vi "Pre_Pic_XY_Basic.vi"() -> ()   [LabVIEW 2011]
uses:
  <vilib>/Utility/miscctls.llb/LVPoint32TypeDef.ctl
  <vilib>/Utility/miscctls.llb/LVBoundsTypeDef.ctl
panel:
  out "mu08txtChoicePicOriginPoint":T1
  out "TxtChoiceBuf":picture
  out "绘图区域大小":T2
  out "Remain":i32
  out "ColorArray":u32[](array[colorbox])=[16770560, 7995178, 2818039]
  out "mbfTxtChoice":bool[](array[boolean])
  out "Index":i32
  out "StrArray":string[](array[string])=["ValveCold", "ValveHot", "ValvePre", "WaterShot", "ValveBleach", "ValveDry", "ValveMist", "ValveSteam", "ValveChange", "ValveSoftener", "ValveFilter", "ValveActiveWash"]
  out "x-y":T3
  in  "TxtChoice_YScrollBar":i32(c297)
  out "TxtChoice":picture
  out "mu08TextOffsetInit":T4={"X_Offset"=0, "Y_Offset"=0, "TxtHigh"=16, "TxtWidth"=111, "TxtInterval"=16}
  out "Vertical":i32=3
  out "Horizontal":i32=92
  out "数值":i32
  in  "Y":i32(c297)
  in  "X":i32(c297)
  out "X_Y坐标系统":picture
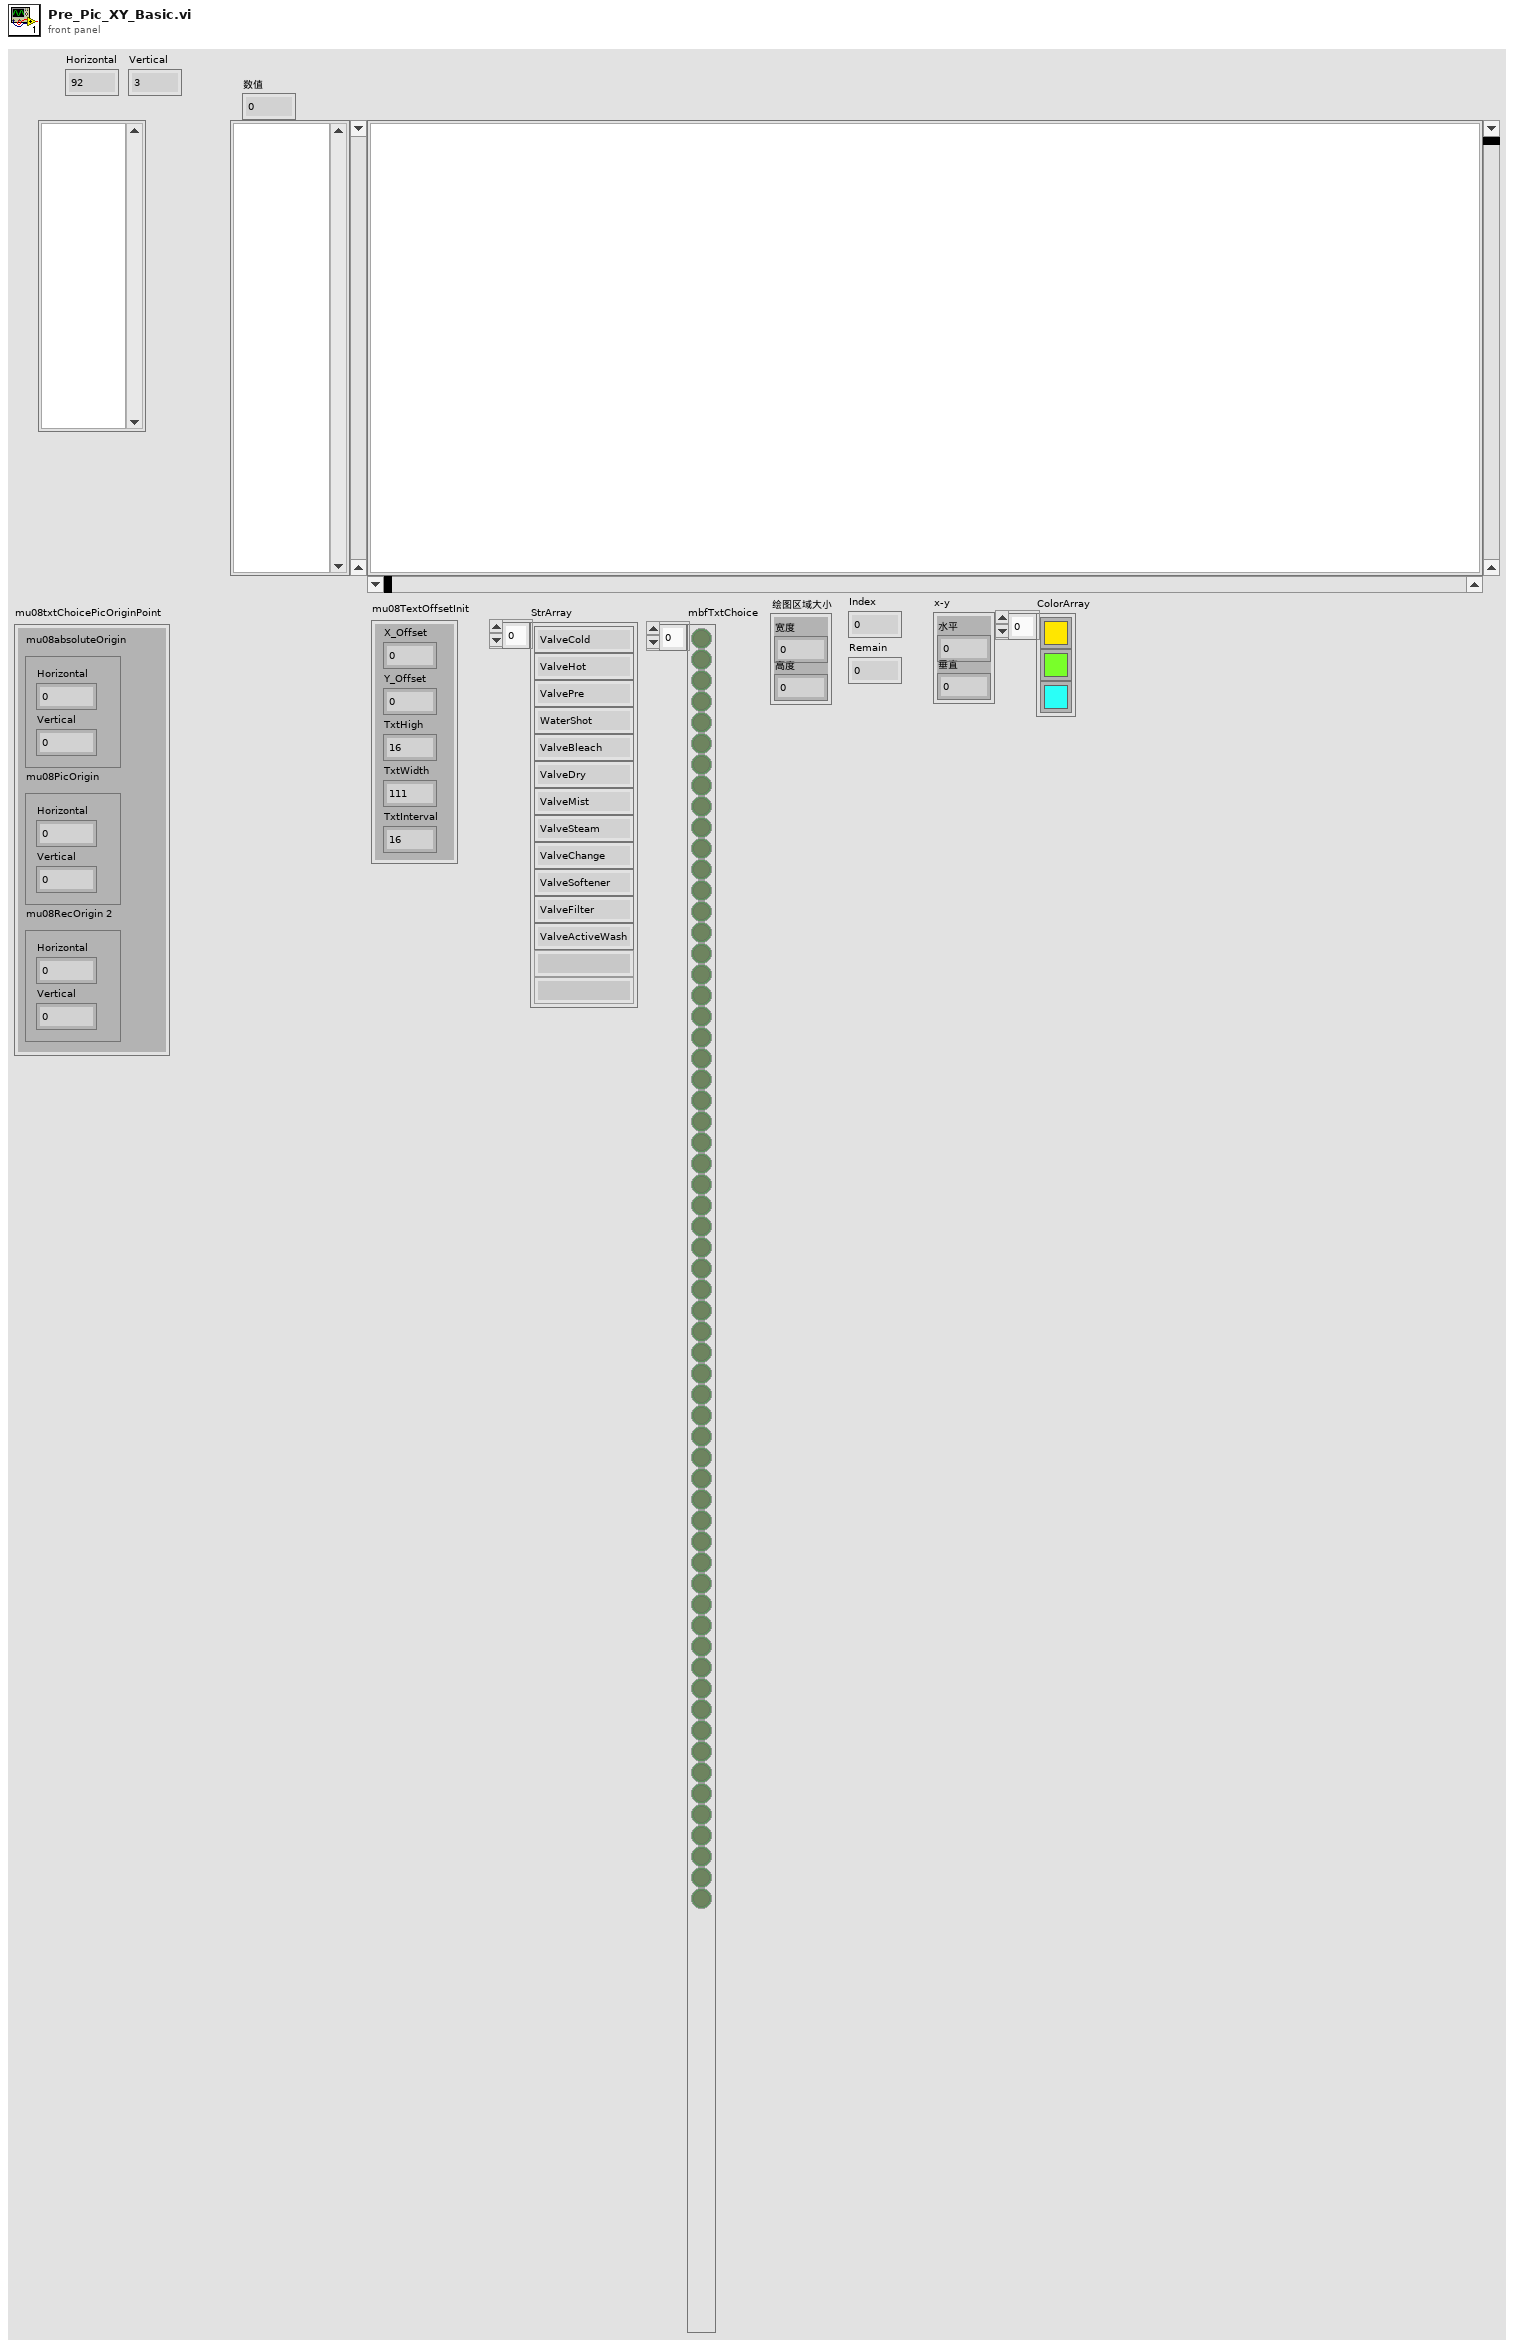
[diagram p1: front panel]
types:
  T1 = cluster{"mu08absoluteOrigin":cluster{"Horizontal":dbl, "Vertical":dbl}, "mu08PicOrigin":cluster{"Horizontal":dbl, "Vertical":dbl}, "mu08RecOrigin 2":cluster{"Horizontal":dbl, "Vertical":dbl}}
  T2 = typedef "LVBoundsTypeDef.ctl" = cluster{"Width":u32, "Height":u32}
  T3 = typedef "LVPoint32TypeDef.ctl" = cluster{"Horizontal":i32, "Vertical":i32}
  T4 = cluster{"X_Offset":u8, "Y_Offset":u8, "TxtHigh":u8, "TxtWidth":u8, "TxtInterval":u8}
  T5 = typedef "LVPositionTypeDef.ctl" = cluster{"Left":i32, "Top":i32}
  T6 = cluster{"Position":T5, cluster{i32, i32}, cluster{i32, i32}}
  T7 = typedef "imagedata.ctl" = cluster{"image type":i32, "image depth":i32, "image":u8[], "mask":u8[], "colors":u32[], "Rectangle":cluster{"left":i16, "top":i16, "right":i16, "bottom":i16}}
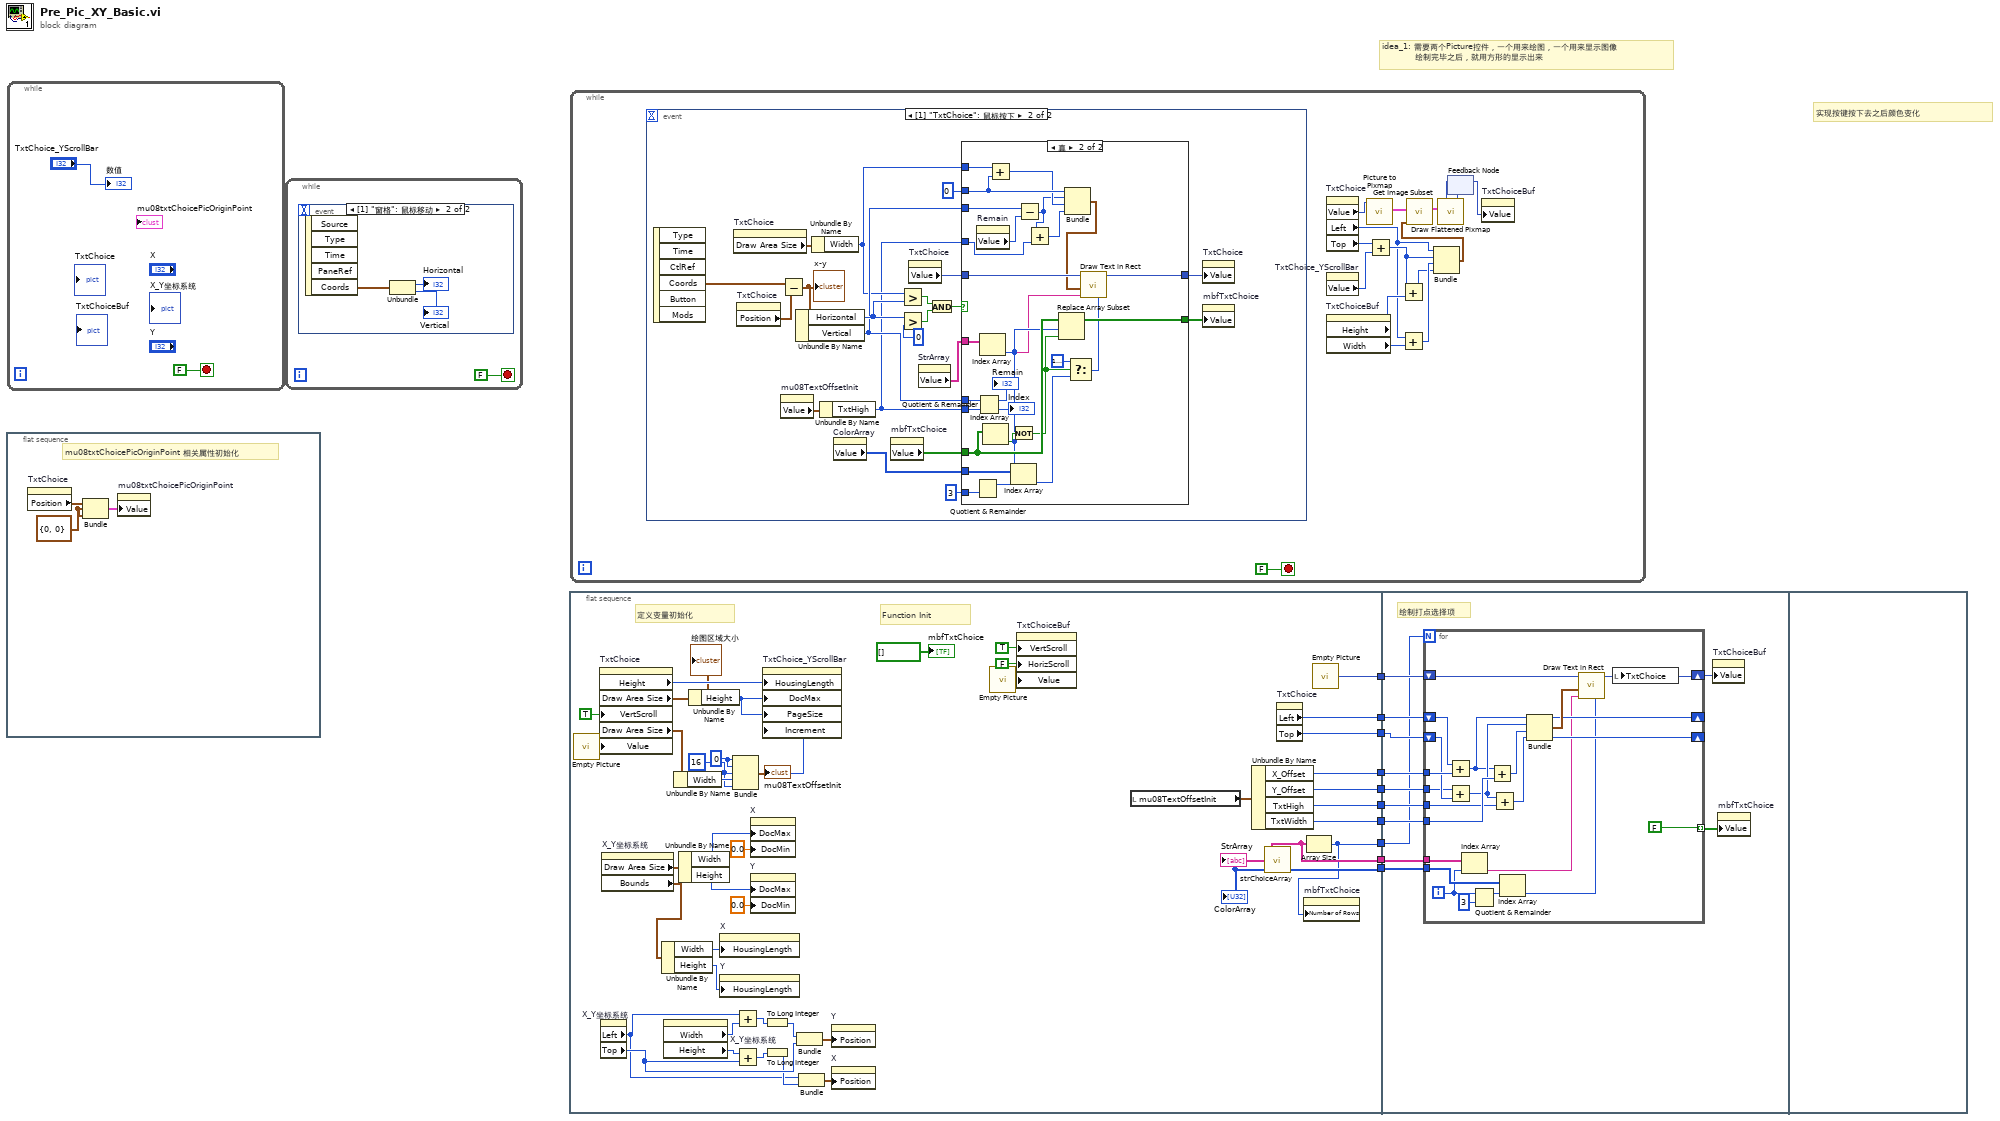
[diagram p0: block diagram]
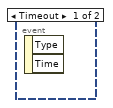
[diagram p2: hidden frame]
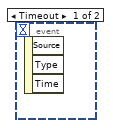
[diagram p4: hidden frame]
diagram:
  # "实现按键按下去之后颜色变化"
  # "idea_1: 需要两个Picture控件，一个用来绘图，一个用来显示图像\n           绘制完毕之后，就用方形的显示出来"
  n1 = flat-sequence {
    frame #0 {
      w12 = cluster{i32, i32} {0, 0}
      # "mu08txtChoicePicOriginPoint 相关属性初始化"
      n2 = property on="TxtChoice" class="Pict"() -> ("Position"=w13:T5)  [unwired: 2 in, 2 out]
      n3 = Bundle("Position"=w13, w12, w12) -> (w11:T6)  [unwired: 1 in]
      n4 = property on="mu08txtChoicePicOriginPoint" class="Clust (严格)"("Value"=w11) -> ()  [unwired: 2 in, 2 out]
    }
  }
  n5 = while {
    stop <- FALSE stop-if-true
    "数值" <- "TxtChoice_YScrollBar"
  }
  n6 = while {
    stop <- FALSE stop-if-true
    n7 = event shown="[1] \"窗格\": 鼠标移动" {
      selector: _ -> [_ _]
      dyn-events: _ -> [_ _]
      timeout: _ -> [_ _]
      event Timeout {
        n8 = event-data() -> ()  [unwired: 1 in, 3 out]
      }
      event Mouse Move {
        n9 = event-data() -> ("Coords"=w19:T3)  [unwired: 1 in, 4 out]
        n10 = Unbundle(w19) -> ("Horizontal"=→"Horizontal":i32, "Vertical"=→"Vertical":i32)
      }
    }
  }
  n11 = flat-sequence {
    tunnel: [w45] -> w10
    tunnel: [w44] -> w9
    tunnel: [w43] -> w8
    tunnel: [w41] -> w7
    tunnel: [w40] -> w6
    tunnel: [w39] -> w5
    tunnel: [w38] -> w4
    tunnel: [w31] -> w3
    tunnel: [w34] -> w2
    tunnel: [w33] -> w1
    tunnel: w10 -> [w74]
    tunnel: w9 -> [w72]
    tunnel: w8 -> [w71]
    tunnel: w7 -> [w73]
    tunnel: w6 -> [w68]
    tunnel: w5 -> [w70]
    tunnel: w4 -> [w69]
    tunnel: w3 -> [w67]
    tunnel: w2 -> [w66]
    tunnel: w1 -> [w65]
    frame #0 {
      w35 = 0
      w23 = 16
      # "Function Init"
      # "定义变量初始化"
      n12 = call "Empty Picture"() -> ("empty picture"=w21:picture)
      n13 = property on="TxtChoice" class="Pict"("VertScroll"=TRUE ("垂直滚动条可见"), "Value"=w21) -> ("Height"=w28:u32, "Draw Area Size"=w27:T2, "Draw Area Size"=w24:T2)  [unwired: 2 in, 2 out]
      "绘图区域大小" <- w27
      n14 = property on="X_Y坐标系统" class="Pict"() -> ("Left"=w49:i32, "Top"=w51:i32)  [unwired: 2 in, 2 out]
      n15 = property on="X_Y坐标系统" class="Pict"() -> ("Draw Area Size"=w62:T2, "Bounds"=w29:T2)  [unwired: 2 in, 2 out]
      n16 = Unbundle By Name(w29) -> ("Width"=w57:u32, "Height"=w56:u32)
      n17 = property on="X_Y坐标系统" class="Pict"() -> ("Width"=w55:u32, "Height"=w54:u32)  [unwired: 2 in, 2 out]
      n18 = Unbundle By Name(w24) -> ("Width"=w37:u32)
      n19 = Unbundle By Name(w62) -> ("Width"=w60:u32, "Height"=w61:u32)
      n20 = Unbundle By Name(w27) -> ("Height"=w26:u32)
      n21 = property on="X" class="Scroll (严格)"("HousingLength"=w57) -> ()  [unwired: 2 in, 2 out]
      n22 = property on="Y" class="Scroll (严格)"("HousingLength"=w56) -> ()  [unwired: 2 in, 2 out]
      n23 = Bundle(w35, w35, w23, "Width"=w37, w23) -> (→"mu08TextOffsetInit":cluster{i32, i32, i32, "Width":u32, i32})  [unwired: 1 in]
      n24 = Add(x=w49, y=w55) -> (x+y=w47:u32)
      n25 = Add(x=w54, y=w51) -> (x+y=w46:u32)
      n26 = property on="X" class="Scroll (严格)"("DocMax"=w60, "DocMin"=0.0 ("滚动范围最小值")) -> ()  [unwired: 2 in, 2 out]
      n27 = property on="Y" class="Scroll (严格)"("DocMax"=w61, "DocMin"=0.0 ("滚动范围最小值")) -> ()  [unwired: 2 in, 2 out]
      n28 = property on="TxtChoice_YScrollBar" class="Scroll (严格)"("HousingLength"=w28, "DocMax"=w26, "PageSize"=w26, "Increment"=w23) -> ()  [unwired: 2 in, 2 out]
      n29 = To Long Integer(number=w47) -> (32bit integer=w53:i32)
      n30 = To Long Integer(number=w46) -> (32bit integer=w50:i32)
      n31 = Bundle(w53, "Top"=w51) -> (w52:cluster{i32, "Top":i32})  [unwired: 1 in]
      n32 = Bundle("Left"=w49, w50) -> (w48:cluster{"Left":i32, i32})  [unwired: 1 in]
      n33 = property on="Y" class="Scroll (严格)"("Position"=w52) -> ()  [unwired: 2 in, 2 out]
      n34 = property on="X" class="Scroll (严格)"("Position"=w48) -> ()  [unwired: 2 in, 2 out]
      n35 = call "Empty Picture"() -> ("empty picture"=w20:picture)
      n36 = property on="TxtChoiceBuf" class="Pict"("VertScroll"=TRUE ("垂直滚动条可见"), "HorizScroll"=FALSE ("水平滚动条可见"), "Value"=w20) -> ()  [unwired: 2 in, 2 out]
      n37 = local read "mu08TextOffsetInit"() -> (w42:T4)
      n38 = Unbundle By Name(w42) -> ("X_Offset"=w41:u8, "Y_Offset"=w40:u8, "TxtHigh"=w38:u8, "TxtWidth"=w39:u8)
      n39 = call "strChoiceArray.vi"() -> ("ColorArray"=w33:u32[], "StrArray"=w34:string[])
      "StrArray" <- w34
      "ColorArray" <- w33
      n40 = property on="TxtChoice" class="Pict"() -> ("Left"=w44:i16, "Top"=w43:i16)  [unwired: 2 in, 2 out]
      n41 = Array Size(array=w34) -> (size(s)=w31:i32)
      n42 = property on="mbfTxtChoice" class="Arr (严格)"("Number of Rows"=w31) -> ()  [unwired: 2 in, 2 out]
      n43 = call "Empty Picture"() -> ("empty picture"=w45:picture)
      "mbfTxtChoice" <- bool[] [] ("mbfTxtChoice")
    }
    frame #1 {
      # "绘制打点选择项"
      n44 = for {
        N: w67 -> [_]
        tunnel: w73 -> [w94]
        tunnel: w70 -> [w91]
        tunnel: w69 -> [w89]
        tunnel: w68 -> [w87]
        shift-right: [w86] -> w63
        shift-left: w74 -> [w95]
        shift-right: [w83] -> _
        shift-left: w72 -> [w93]
        shift-right: [w84] -> _
        shift-left: w71 -> [w92]
        tunnel: w66 -> [w82]
        tunnel: w65 -> [w80]
        tunnel: [FALSE] -> w64 mode=indexing
        i -> [w79]
        n45 = Add(x=w93, y=w94) -> (x+y=w83:i16)
        n46 = Add(x=w87, y=w92) -> (x+y=w85:i16)
        n47 = Index Array(array=w82, index=w79) -> (element=w81:string)
        n48 = Quotient & Remainder(x=w79, y=3) -> (x-y*floor(x/y)=w77:i32)  [unwired: 1 out]
        n49 = Add(x=w83, y=w91) -> (x+y=w90:i16)
        n50 = Add(x=w85, y=w89) -> (x+y=w84:i16)
        n51 = Index Array(array=w80, index=w77) -> (element=w76:u32)
        n52 = Bundle(w83, w85, w90, w84) -> (w88:cluster{i16, i16, i16, i16})  [unwired: 1 in]
        n53 = call <vilib>:"Draw Text in Rect.vi"("BG color(transparent)"=w76, "text"=w81, "rect"=w88, "picture"=w95) -> ("new picture"=w86:picture)  [unwired: 7 in]
        n54 = local write "TxtChoice"(w86) -> ()
      }
      n55 = property on="TxtChoiceBuf" class="Pict"("Value"=w63) -> ()  [unwired: 2 in, 2 out]
      n56 = property on="mbfTxtChoice" class="Arr (严格)"("Value"=w64) -> ()  [unwired: 2 in, 2 out]
    }
    frame #2 {
    }
  }
  n57 = while {
    stop <- FALSE stop-if-true
    n58 = event shown="[1] \"TxtChoice\": 鼠标按下" {
      selector: _ -> [_ _]
      dyn-events: _ -> [_ _]
      timeout: _ -> [_ _]
      event Timeout {
        n59 = event-data() -> ()  [unwired: 1 in, 2 out]
      }
      event "TxtChoice": Mouse Down {
        n60 = event-data() -> ("Coords"=w131:T3)  [unwired: 1 in, 5 out]
        n61 = property on="TxtChoice" class="Pict"() -> ("Draw Area Size"=w126:T2)  [unwired: 2 in, 2 out]
        n62 = property on="TxtChoice" class="Pict"() -> ("Position"=w130:T5)  [unwired: 2 in, 2 out]
        n63 = Subtract(x=w131, y=w130) -> (x-y=w129:T3)
        "x-y" <- w129
        n64 = property on="mu08TextOffsetInit" class="Clust (严格)"() -> ("Value"=w122:T4)  [unwired: 2 in, 2 out]
        n65 = Unbundle By Name(w129) -> ("Horizontal"=w127:i32, "Vertical"=w113:i32)
        n66 = Unbundle By Name(w126) -> ("Width"=w112:u32)
        n67 = Unbundle By Name(w122) -> ("TxtHigh"=w111:u8)
        n68 = property on="ColorArray" class="Arr (严格)"() -> ("Value"=w116:u32[])  [unwired: 2 in, 2 out]
        n69 = property on="mbfTxtChoice" class="Arr (严格)"() -> ("Value"=w118:bool[])  [unwired: 2 in, 2 out]
        n70 = Greater?(x=w112, y=w127) -> (0:w125:bool)
        n71 = Greater?(x=w127, y=0) -> (0:w124:bool)
        n72 = property on="TxtChoice" class="Pict"() -> ("Value"=w121:picture)  [unwired: 2 in, 2 out]
        n73 = property on="StrArray" class="Arr (严格)"() -> ("Value"=w119:string[])  [unwired: 2 in, 2 out]
        n74 = And(x=w125, y=w124) -> (x .and. y?=w123:bool)
        n75 = case shown="真" w123 {
          tunnel: w113 -> [_ w160]
          tunnel: w111 -> [_ w159]
          tunnel: w121 -> [w133 w158]
          tunnel: [w133 w157] -> w120
          tunnel: w119 -> [_ w156]
          tunnel: w118 -> [w132 w155]
          tunnel: [w132 w153] -> w117
          tunnel: w116 -> [_ w152]
          tunnel: 3 -> [_ w151]
          tunnel: 0 -> [_ w143]
          tunnel: w113 -> [_ w141]
          tunnel: w112 -> [_ w140]
          tunnel: w111 -> [_ w137]
          frame False {
          }
          frame True {
            n76 = property on="Remain" class="DigNum (严格)"() -> ("Value"=w142:i32)  [unwired: 2 in, 2 out]
            n77 = Quotient & Remainder(x=w160, y=w159) -> (x-y*floor(x/y)=→"Remain":i32, floor(x/y)=w147:i32)
            "Index" <- w147
            n78 = Quotient & Remainder(x=w147, y=w151) -> (x-y*floor(x/y)=w134:i32)  [unwired: 1 out]
            n79 = Index Array(array=w156, index=w147) -> (element=w146:string)
            n80 = Index Array(array=w155, index=w147) -> (element=w154:bool)
            n81 = Add(x=w140, y=w143) -> (x+y=w139:u32)
            n82 = Not(x=w154) -> (.not. x?=w150:bool)
            n83 = Index Array(array=w152, index=w134) -> (element=w148:u32)
            n84 = Subtract(x=w141, y=w142) -> (x-y=w138:i32)
            n85 = Add(x=w138, y=w137) -> (x+y=w136:i32)
            n86 = Replace Array Subset(array=w155, new element=w150, index=w147) -> (w153:bool[])
            n87 = Bundle(w143, w138, w139, w136) -> (w135:cluster{i32, i32, u32, i32})  [unwired: 1 in]
            n88 = Select(t=u32 16777226 ("BG color(transparent)"), s=w150, f=w148) -> (s? t:f=w145:u32)
            n89 = call <vilib>:"Draw Text in Rect.vi"("BG color(transparent)"=w145, "text"=w146, "rect"=w135, "picture"=w158) -> ("new picture"=w157:picture)  [unwired: 7 in]
          }
        }
        n90 = property on="TxtChoice" class="Pict"("Value"=w120) -> ()  [unwired: 2 in, 2 out]
        n91 = property on="mbfTxtChoice" class="Arr (严格)"("Value"=w117) -> ()  [unwired: 2 in, 2 out]
      }
    }
    n92 = property on="TxtChoice" class="Pict"() -> ("Value"=w103:picture, "Left"=w96:i16, "Top"=w100:i16)  [unwired: 2 in, 2 out]
    n93 = property on="TxtChoice_YScrollBar" class="Scroll (严格)"() -> ("Value"=w99:i32)  [unwired: 2 in, 2 out]
    n94 = property on="TxtChoiceBuf" class="Pict"() -> ("Height"=w106:u32, "Width"=w97:u32)  [unwired: 2 in, 2 out]
    n95 = call <vilib>:"Picture to Pixmap.vi"("picture"=w103) -> ("image data"=w109:T7)  [unwired: 9 in, 1 out]
    n96 = Add(x=w100, y=w99) -> (x+y=w105:i32)
    n97 = Add(x=w105, y=w106) -> (x+y=w104:u32)
    n98 = Add(x=w96, y=w97) -> (x+y=w107:u32)
    n99 = Bundle("Left"=w96, w105, w107, w104) -> (w98:cluster{"Left":i16, i32, u32, u32})  [unwired: 1 in]
    n100 = call <vilib>:"Get Image Subset.vi"("subset rect"=w98, "image data"=w109) -> ("image subset"=w108:T7)  [unwired: 4 in, 1 out]
    n101 = feedback #1() -> (w101:picture)  [unwired: 1 in]
    n102 = call <vilib>:"Draw Flattened Pixmap.vi"("image data"=w108, "picture"=w101) -> ("new picture"=w102:picture)  [unwired: 7 in]
    n103 = feedback-in #1(w102) -> ()
    n104 = property on="TxtChoiceBuf" class="Pict"("Value"=w101) -> ()  [unwired: 2 in, 2 out]
  }
